vi "ftt& target Color Display.vi"(8 "error in (no error)":errorcluster, 9 "Tatget":string, 10 "ftt":string, 11 "Cluster":T4) -> (0 "error out":errorcluster)   [LabVIEW 2014]
uses:
  Type'def/CN image Ctr.ctl
  <vilib>/picture/picture.llb/imagedata.ctl
  Type'def/CN Config Ctr.ctl
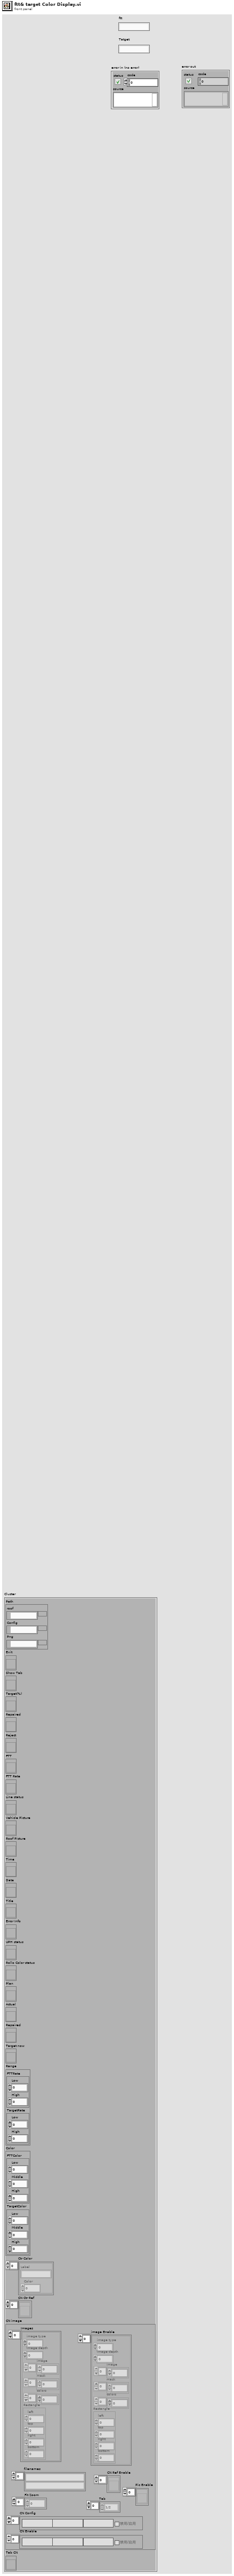
[diagram p1: front panel]
types:
  T1 = typedef "CN image Ctr.ctl" = cluster{"Images":T2[], "filenames":string[], "Fit Zoom":dbl[], "CN Config":T3[], "CN Enable":T3[], "image Enable":T2[], "CN Ref Enable":refnum<vi>[], "Tab ":enum32{"1/2", "1/3", "1/4", "1/5", "2/5", "3/5"}[], "Pic Enable":refnum<vi>[]}
  T2 = typedef "imagedata.ctl" = cluster{"image type":i32, "image depth":i32, "image":u8[], "mask":u8[], "colors":u32[], "Rectangle":cluster{"left":i16, "top":i16, "right":i16, "bottom":i16}}
  T3 = typedef "CN Config Ctr.ctl" = cluster{"Model":string, "Pic_Name":string, "CarName":string, "En/Disable":bool}
  T4 = cluster{"Path":cluster{"roof":path, "Config":path, "Png":path}, "Exit":refnum<vi>, "Show Tab":refnum<vi>, "Target(%)":refnum<vi>, "Repaired":refnum<vi>, "Reject":refnum<vi>, "FTT":refnum<vi>, "FTT Rate":refnum<vi>, "Line status":refnum<vi>, "Vehicle Picture":refnum<vi>, "Roof Picture":refnum<vi>, "Time":refnum<vi>, "Date":refnum<vi>, "Title":refnum<vi>, "Error Info":refnum<vi>, "UPH status":refnum<vi>, "Rollo Color status":refnum<vi>, "Plan":refnum<vi>, "Actual":refnum<vi>, "Repaired":refnum<vi>, "Target now":refnum<vi>, "Range":cluster{"FTTRate":cluster{"Low":u32, "High":u32}, "TargetRate":cluster{"Low":u32, "High":u32}}, "Color":cluster{"FTTColor":cluster{"Low":u32, "Middle":u32, "High":u32}, "TargetColor":cluster{"Low":u32, "Middle":u32, "High":u32}}, "Ctr Color":cluster{"Label":string, "Color":u32}[], "CN Ctr Ref":refnum<vi>[], "CN image":T1, "Tab CN":refnum<vi>}
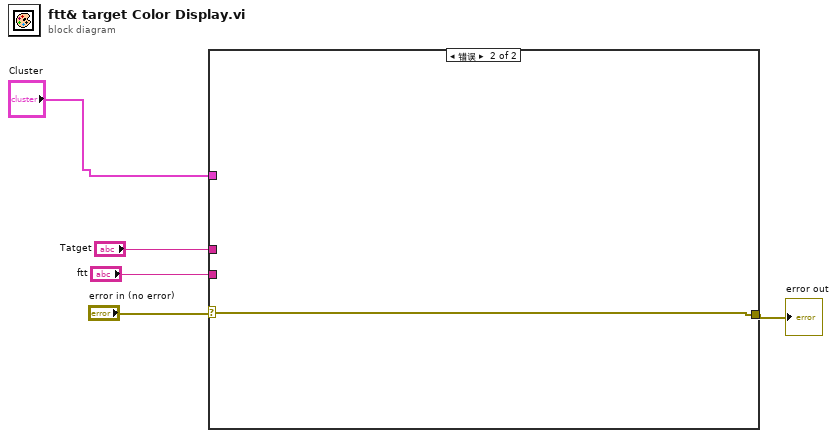
[diagram p0: block diagram]
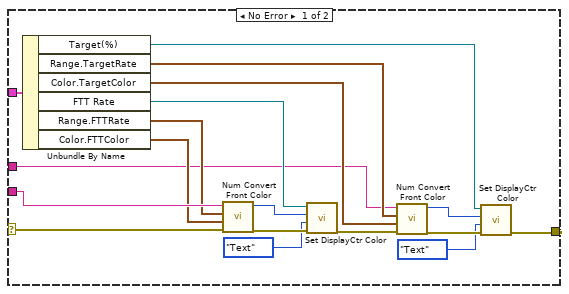
[diagram p2: hidden frame]
diagram:
  n1 = case shown="错误" "error in (no error)" {
    selector: "error in (no error)" -> [w23 w24]
    tunnel: "ftt" -> [w22 _]
    tunnel: "Cluster" -> [w21 _]
    tunnel: "Tatget" -> [w8 _]
    tunnel: [w6 w24] -> w2
    frame No Error {
      n2 = Unbundle By Name(w21) -> ("Target(%)"=w7:refnum<vi>, "Range.TargetRate"=w10:cluster{"Low":u32, "High":u32}, "Color.TargetColor"=w9:cluster{"Low":u32, "Middle":u32, "High":u32}, "FTT Rate"=w16:refnum<vi>, "Range.FTTRate"=w20:cluster{"Low":u32, "High":u32}, "Color.FTTColor"=w19:cluster{"Low":u32, "Middle":u32, "High":u32})
      n3 = call "Num Convert Front Color.vi"("error in (no error)"=w23, "FTTColor"=w19, "TargetRate"=w20, "FTT Rate"=w22) -> ("error out"=w18:errorcluster, "Middle"=w17:u32)  [unwired: 6 in]
      n4 = call "Set DisplayCtr Color.vi"("error in (no error)"=w18, "Mode"=enum16{"Label", "Caption", "Text"}."Text", "Color Box"=w17, "Ctr Ref"=w16) -> ("error IO"=w11:errorcluster)  [unwired: 7 in]
      n5 = call "Num Convert Front Color.vi"("error in (no error)"=w11, "FTTColor"=w9, "TargetRate"=w10, "FTT Rate"=w8) -> ("error out"=w14:errorcluster, "Middle"=w13:u32)  [unwired: 6 in]
      n6 = call "Set DisplayCtr Color.vi"("error in (no error)"=w14, "Mode"=enum16{"Label", "Caption", "Text"}."Text", "Color Box"=w13, "Ctr Ref"=w7) -> ("error IO"=w6:errorcluster)  [unwired: 7 in]
    }
    frame Error {
    }
  }
  "error out" <- w2
